vi "DigitalOutputCommand.vi"(1 "FPGA I/O In":refnum<k21>="Slot6/CH0") -> ()   [LabVIEW 2019]
uses:
  <vilib>/rvi/interface/RandomDataEmulation/niFpgaRandomDataHandleErrors.vi
  <vilib>/rvi/eio/common/nirviEmuTemplateMethod_errors.vi
  <vilib>/rvi/DataTransferAndStorage/Container/XNode/niFpgaContainer.xnode
  <vilib>/rvi/interface/RandomDataEmulation/nirviRandomDataFpgaReadWriteTemplate.vi
  <vilib>/eio/EIONode/EIONode.xnode
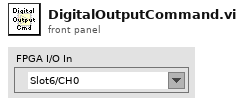
[diagram p1: front panel]
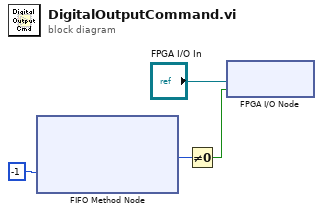
[diagram p0: block diagram]
diagram:
  n1 = xnode ("FIFO Method Node")("Timeout"=-1) -> ("Element"=w2:u16)  [unwired: 1 in, 2 out]
  n2 = Not Equal To 0?(x=w2) -> (x != 0?=w1:bool)
  n3 = xnode "FPGA I/O Node"("I/O Item"=w1, "FPGA I/O In"="FPGA I/O In") -> ()  [unwired: 1 out]
